vi "DataLog Linearly Interpolate Between.vi"(1 "at":dbl format="%<%H:%M:%S%2u\n%Y/%m/%d>T", 2 "point 2":T1 {"value" format="%.3e"; "time" format="%<%H:%M:%S%2u\n%Y/%m/%d>T"}, 3 "point 1":T1 {"value" format="%.3e"; "time" format="%<%H:%M:%S%2u\n%Y/%m/%d>T"}) -> (0 "value":dbl format="%.2f")   [LabVIEW 2012]
doc: "Do a linear interpolation between two points given a time at which to interpolate. Takes into account the corner case where the time is at one point and the other point has a NaN value. In such a case, no interpolation is done to avoid erroneously returning NaN. The times of two points should not be identical or else this function will divide by zero."
uses:
  typedefs/clusters/t_DataLog Point.ctl
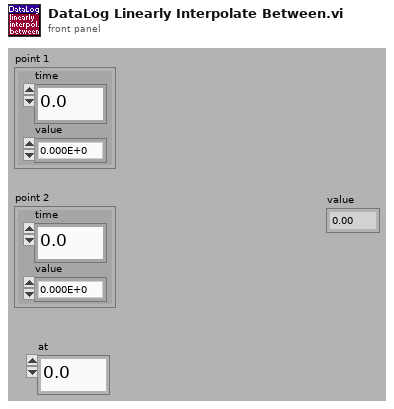
[diagram p1: front panel]
types:
  T1 = typedef "t_DataLog Point.ctl" = cluster{"time":dbl, "value":dbl}
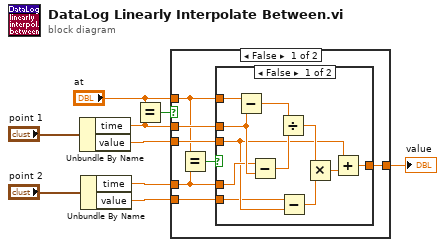
[diagram p0: block diagram]
diagram:
  n1 = Unbundle By Name("point 1") -> ("time"=w2:dbl, "value"=w6:dbl)
  n2 = Unbundle By Name("point 2") -> ("time"=w9:dbl, "value"=w5:dbl)
  n3 = Equal?(x="at", y=w2) -> (x = y?=w1:bool)
  n4 = case shown="False" w1 {
    tunnel: w2 -> [w16 _]
    tunnel: w9 -> [w11 _]
    tunnel: "at" -> [w10 _]
    tunnel: w6 -> [w15 w29]
    tunnel: w5 -> [w14 _]
    tunnel: [w13 w29] -> w4
    frame False {
      n5 = Equal?(x=w10, y=w11) -> (x = y?=w12:bool)
      n6 = case shown="False" w12 {
        tunnel: w16 -> [w24 _]
        tunnel: w11 -> [w23 _]
        tunnel: w10 -> [w22 _]
        tunnel: w15 -> [w21 _]
        tunnel: w14 -> [w18 w28]
        tunnel: [w17 w28] -> w13
        frame False {
          n7 = Subtract(x=w22, y=w24) -> (x-y=w20:dbl)
          n8 = Subtract(x=w23, y=w24) -> (x-y=w25:dbl)
          n9 = Divide(x=w20, y=w25) -> (x/y=w26:dbl)
          n10 = Subtract(x=w18, y=w21) -> (x-y=w19:dbl)
          n11 = Multiply(x=w26, y=w19) -> (x*y=w27:dbl)
          n12 = Add(x=w21, y=w27) -> (x+y=w17:dbl)
        }
        frame True {
          # "Required to make value\ninsensitive to NaN in\nfirst point when\ninterpolation time at\nsecond point."
        }
      }
    }
    frame True {
      # "Required to make value\ninsensitive to NaN in\nsecond point when\ninterpolation time at\nfirst point."
    }
  }
  "value" <- w4
